vi "String to I16.vi"(8 "error in":errorcluster, 11 "String":string) -> (0 "error out":errorcluster, 3 "I16":i16)   [LabVIEW 2024, in "Electronic Datasheet.lvlib"]
doc: "Converts the string representation of a number in a specified base to an equivalent 32-bit signed integer."
uses:
  Electronic Datasheet.lvlib
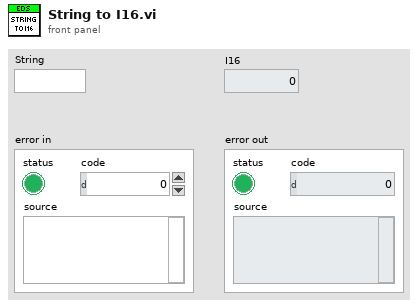
[diagram p1: front panel]
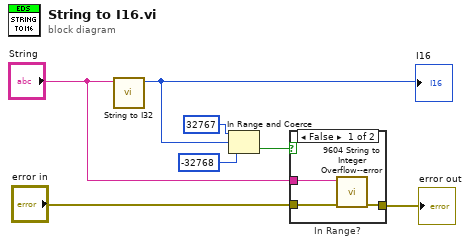
[diagram p0: block diagram]
diagram:
  n1 = call "String to I32.vi"("String"="String") -> ("I32"=w5:i32)  [unwired: 10 in]
  "I16" <- w5
  n2 = In Range and Coerce(upper limit=32767, x=w5, lower limit=-32768 ("upper limit")) -> (In Range?=w4:bool)  [unwired: 1 out]
  n3 = case "In Range?" shown="False" w4 {
    tunnel: "error in" -> [w10 w11]
    tunnel: [w9 w11] -> w2
    tunnel: "String" -> [w8 _]
    frame False {
      n4 = call "9604 String to Integer Overflow--error.vi"("error in"=w10, "Integer String"=w8) -> ("error out"=w9:errorcluster)  [unwired: 9 in]
    }
    frame True {
    }
  }
  "error out" <- w2
